vi "ClusterToAttrMap.vi"(4 "Recursive?(T)":bool=TRUE, 8 "error in (no error)":errorcluster, 11 "data":variant) -> (0 "error out":errorcluster, 3 "AttrMap":T1)   [LabVIEW 2019, in "lv-apt-json-file.lvlib"]
uses:
  lv-apt-json-file.lvlib
  Def-AttrMap.ctl
  _Support/AttrMap-SetValue-CORE.vi/6e91e2cf-a420-477d-bf86-627245081caf.vi
  _Support/AttrMap-UnpackNameMap.vi
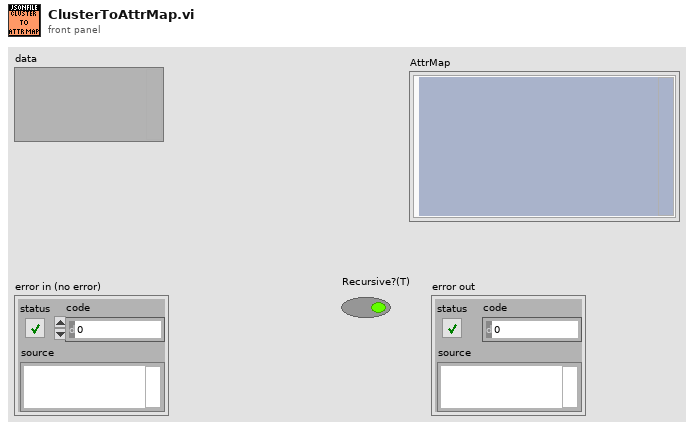
[diagram p1: front panel]
types:
  T1 = typedef "lv-apt-json-file.lvlib/Def-AttrMap.ctl" = cluster{"Map":variant}
  T2 = typedef "Type Descriptor Enumeration__ogtk.ctl" = enum8{"<Null>", "I8", "I16", "I32", "I64", "U8", "U16", "U32", "U64", "SGL", "DBL", "EXT", "CSG", "CDB", "CXT", "0x0F", "0x10", "0x11", "0x12", "0x13", "0x14", "Enum U8", "Enum U16", "Enum U32", "Enum U64", "SGL PQ", "DBL PQ", "EXT PQ", "CSG PQ", "CDB PQ", "CXT PQ", "0x1F", "0x20", "Boolean", "0x22", "0x23", "0x24", "0x25", "0x26", "0x27", "0x28", "0x29", "0x2A", "0x2B", "0x2C", "0x2D", "0x2E", "0x2F", "String", "0x31", "Path", "Pict", "0x34", "0x35", "0x36", "DAQ", "0x38", "0x39", "0x3A", "0x3B", "0x3C", "0x3D", "0x3E", "0x3F", "Array", "0x41", "0x42", "0x43", "0x44", "0x45", "0x46", "0x47", "0x48", "0x49", "0x4A", "0x4B", "0x4C", "0x4D", "0x4E", "0x4F", "Cluster", "0x51", "0x52", "Variant", "Waveform", "0x55", "0x56", "0x57", "0x58", "0x59", "0x5A", "0x5B", "0x5C", "0x5D", "0x5E", "0x5F", "0x60", "0x61", "0x62", "0x63", "0x64", "0x65", "0x66", "0x67", "0x68", "0x69", "0x6A", "0x6B", "0x6C", "0x6D", "0x6E", "0x6F", "Refnum"}
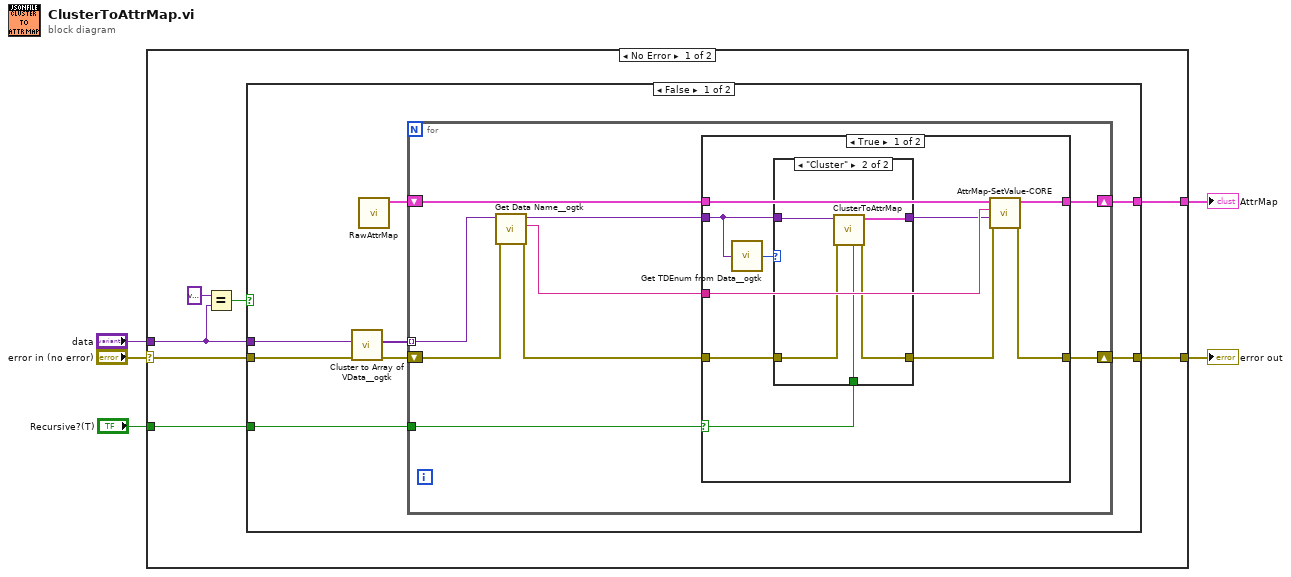
[diagram p0: block diagram]
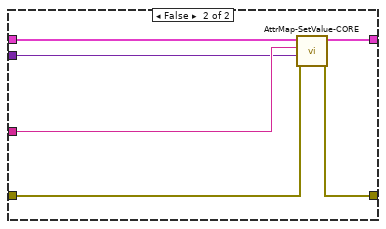
[diagram p3: hidden frame]
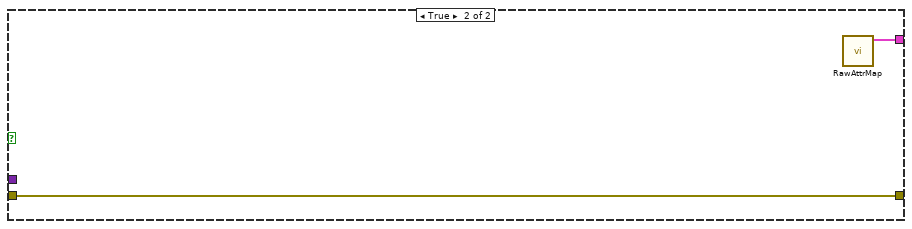
[diagram p4: hidden frame]
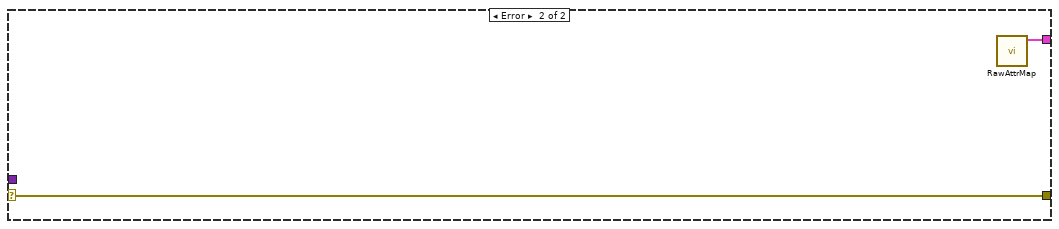
[diagram p5: hidden frame]
diagram:
  n1 = case shown="No Error" "error in (no error)" {
    selector: "error in (no error)" -> [w10 w56]
    tunnel: [w12 w55] -> w5
    tunnel: [w11 w56] -> w4
    tunnel: "data" -> [w8 _]
    tunnel: "Recursive?(T)" -> [w6 _]
    frame No Error {
      n2 = Equal?(x=variant, y=w8) -> (x = y?=w7:bool)
      n3 = case shown="False" w7 {
        tunnel: [w20 w53] -> w12
        tunnel: [w19 w54] -> w11
        tunnel: w10 -> [w18 w54]
        tunnel: w8 -> [w15 _]
        tunnel: w6 -> [w13 _]
        frame False {
          n4 = call <userlib>:"Cluster to Array of VData__ogtk.vi"("error in (no error)"=w18, "Cluster"=w15) -> ("error out"=w17:errorcluster, "Array of VData"=w16:variant[])  [unwired: 8 in]
          n5 = call "RawAttrMap.vi"() -> ("AttrMap"=w14:T1)  [unwired: 11 in]
          n6 = for {
            tunnel: w16 -> [w24] mode=indexing
            shift-right: [w28] -> w20
            shift-left: w14 -> [w29]
            shift-right: [w27] -> w19
            shift-left: w17 -> [w26]
            tunnel: w13 -> [w21]
            n7 = call <userlib>:"Get Data Name__ogtk.vi"("error in (no error)"=w26, "Data"=w24) -> ("error out"=w22:errorcluster, "Data Name"=w25:string, "Data dup"=w23:variant)  [unwired: 7 in]
            n8 = case shown="True" w21 {
              selector: w21 -> [w30 _]
              tunnel: w29 -> [w39 w52]
              tunnel: [w38 w51] -> w28
              tunnel: [w37 w50] -> w27
              tunnel: w25 -> [w36 w49]
              tunnel: w23 -> [w33 w48]
              tunnel: w22 -> [w32 w47]
              frame True {
                n9 = call <userlib>:"Get TDEnum from Data__ogtk.vi"("Data"=w33) -> ("Type Descriptor Enumeration"=w35:T2)  [unwired: 4 in]
                n10 = case shown="\"Cluster\"" w35 {
                  tunnel: [w41 w45] -> w34
                  tunnel: w33 -> [w41 w46]
                  tunnel: [w40 w44] -> w31
                  tunnel: w32 -> [w40 w43]
                  tunnel: w30 -> [_ w42]
                  frame Default {
                  }
                  frame "Cluster" {
                    n11 = call "ClusterToAttrMap.vi"("Recursive?(T)"=w42, "error in (no error)"=w43, "data"=w46) -> ("error out"=w44:errorcluster, "AttrMap"=w45:T1)  [unwired: 7 in]
                  }
                }
                n12 = call "AttrMap-SetValue-CORE.vi"("error in (no error)"=w31, "Value"=w34, "Key"=w36, "AttrMap in"=w39) -> ("error out"=w37:errorcluster, "AttrMap out"=w38:T1)  [unwired: 5 in, 1 out]
              }
              frame False {
                n13 = call "AttrMap-SetValue-CORE.vi"("error in (no error)"=w47, "Value"=w48, "Key"=w49, "AttrMap in"=w52) -> ("error out"=w50:errorcluster, "AttrMap out"=w51:T1)  [unwired: 5 in, 1 out]
              }
            }
          }
        }
        frame True {
          n14 = call "RawAttrMap.vi"() -> ("AttrMap"=w53:T1)  [unwired: 11 in]
        }
      }
    }
    frame Error {
      n15 = call "RawAttrMap.vi"() -> ("AttrMap"=w55:T1)  [unwired: 11 in]
    }
  }
  "AttrMap" <- w5
  "error out" <- w4
